vi "MoveSinglePIMotor.vi"(0 "System no.":i32=1 min=1 step=1, 1 "Axes to move":string[](array[string]), 2 "Move":dbl[](array[numeric]) format="%.6f", 5 "error in":errorcluster, 6 "Define home":bool, 7 "Move relative (-)":bool, 8 "Go home":bool, 9 "Move relative (+)":bool, 11 "Move absolute":bool, 12 "Stop refnum":refnum<vi>) -> (15 "Position":dbl[](array[numeric]) format="%.6f", 19 "error out":errorcluster)   [LabVIEW 2014]
doc: "This VI is runs in a loop until the stop button is pressed, the stop reference is TRUE or an error occures. It lets the operator set the velocity, move the connected axes to relative, absolute or to the home position, and reads the current position continuosly. The diagram shows how to combine the driver and support VIs for these tasks. Use the Help?Show Context Help menu sequence in the LabVIEW environment to display the Context Help window with the VI and control/indicator descriptions.\nRun \" XXXX_Configuration_Setup.vi\" (with XXXX being the PI product number of your system) prior to running this VI. \n\nValid for: C-843, C-843.PM, C-865, C-866, Mercury"
uses:
  C:/Users/Public/PI/GCSMergedLabVIEW/Low Level/General command.llb/Global2 (Array).vi
panel:
  in  "Clear":bool
  in  "stop":bool
  out "Conn. Axes":string[](array[string])
  # "Command move:"
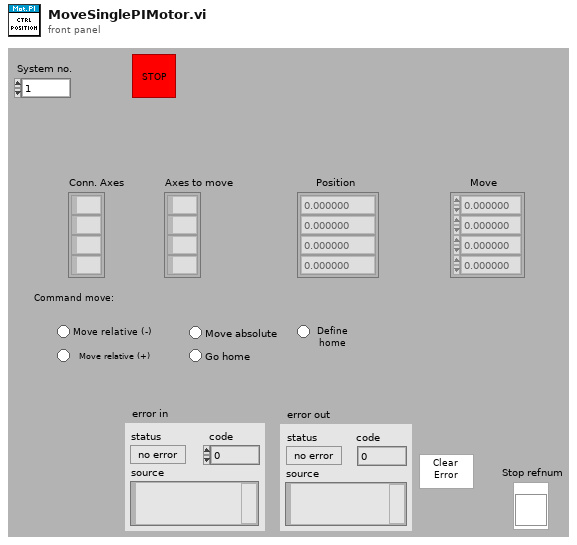
[diagram p1: front panel]
types:
  T1 = typedef "Controller names.ctl" = enum16{"None", "Analog", "C-702", "C-843", "C-843.PM", "C-844", "C-848", "C-865", "C-866", "C-867", "C-880", "C-884", "E-516", "E-517", "E-709", "E-710", "E-712", "E-725", "E-753", "E-755", "E-761", "E-816", "E-861", "E-870", "F-206", "HydraPollux", "M-840", "M-850", "M-8X0", "Mercury", "Mercury_GCS"}
  T2 = cluster{"Conn. axes":string[], "Controller name":T1}[]
  T3 = cluster{"Conn. axes":string[], "Controller name":T1}
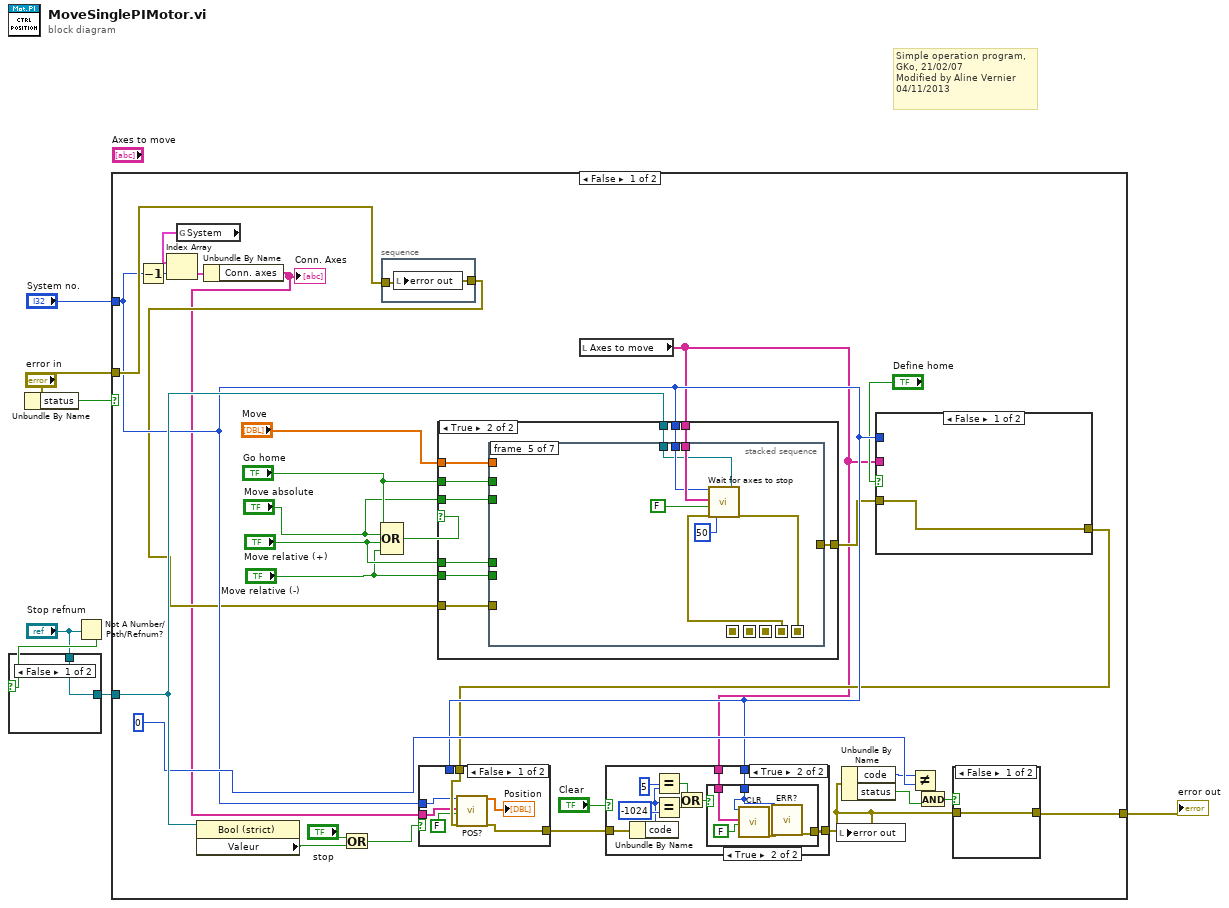
[diagram p0: block diagram]
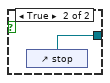
[diagram p2: hidden frame]
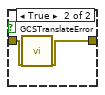
[diagram p3: hidden frame]
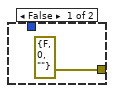
[diagram p5: hidden frame]
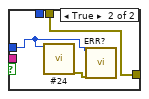
[diagram p6: hidden frame]
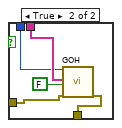
[diagram p9: hidden frame]
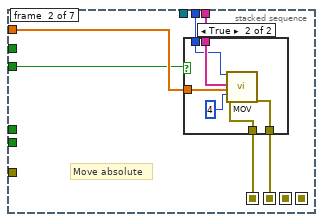
[diagram p10: hidden frame]
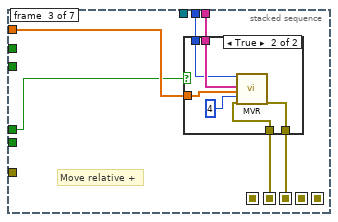
[diagram p12: hidden frame]
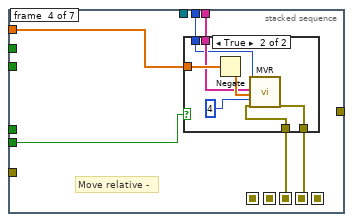
[diagram p14: hidden frame]
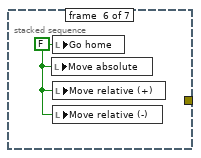
[diagram p16: hidden frame]
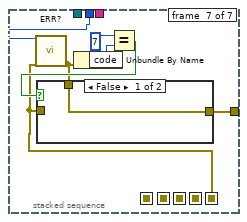
[diagram p17: hidden frame]
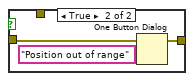
[diagram p18: hidden frame]
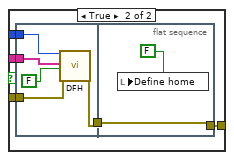
[diagram p19: hidden frame]
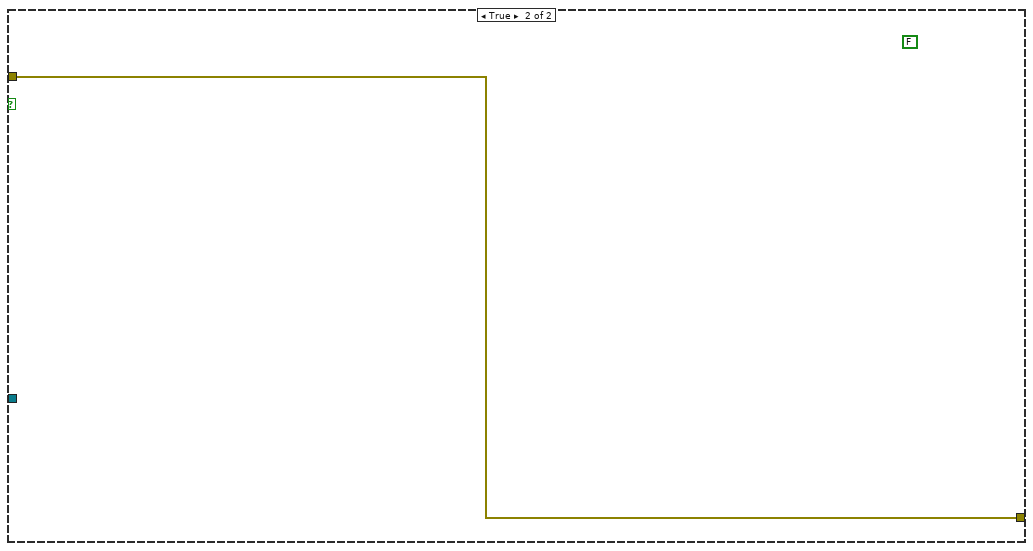
[diagram p20: hidden frame]
diagram:
  # "Simple operation program,\nGKo, 21/02/07\nModified by Aline Vernier\n04/11/2013"
  n1 = Unbundle By Name("error in") -> ("status"=w6:bool)
  n2 = Not A Number/Path/Refnum?(number/path/refnum="Stop refnum") -> (NaN/Path/Refnum?=w3:bool)
  n3 = case shown="False" w3 {
    tunnel: [w8 w9] -> w2
    tunnel: "Stop refnum" -> [w8 _]
    frame False {
    }
    frame True {
      n4 = control-ref of="stop"() -> (w9:refnum<vi>)
    }
  }
  n5 = case shown="False" w6 {
    tunnel: [w39 w163] -> w5
    tunnel: "error in" -> [w38 w163]
    tunnel: "System no." -> [w35 _]
    tunnel: w2 -> [w37 _]
    frame False {
      n6 = Decrement(x=w35) -> (x-1=w34:i32)
      n7 = global read "Global2 (Array).vi" "System"() -> (w33:T2)
      n8 = Index Array(array=w33, index=w34) -> (element=w32:T3)
      n9 = property class="Bool (strict)"(reference=w37) -> ("Valeur"=w26:bool)  [unwired: 1 in, 2 out]
      n10 = Unbundle By Name(w32) -> ("Conn. axes"=w11:string[])
      "Conn. Axes" <- w11
      n11 = Or(x="stop", y=w26) -> (x .or. y?=w12:bool)
      n12 = Compound Arithmetic op=OR("Go home", "Move absolute", "Move relative (+)", "Move relative (-)") -> (w14:bool)
      n13 = stacked-sequence {
        tunnel: w38 -> [w162]
        tunnel: [w162] -> w31
        frame #0 {
          n14 = local write "error out"(w162) -> ()
        }
      }
      n15 = local read "Axes to move"() -> (w13:string[])
      n16 = case shown="True" w14 {
        tunnel: "Go home" -> [_ w79]
        tunnel: w35 -> [_ w78]
        tunnel: w13 -> [_ w77]
        tunnel: "Move" -> [_ w76]
        tunnel: [w69 w75] -> w25
        tunnel: w37 -> [_ w74]
        tunnel: "Move absolute" -> [_ w73]
        tunnel: "Move relative (+)" -> [_ w72]
        tunnel: w31 -> [w69 w71]
        tunnel: "Move relative (-)" -> [_ w70]
        frame False {
        }
        frame True {
          n17 = stacked-sequence {
            seq-local: [w81 _ _ _ _ _ _] -> [_ w94 _ _ _ _ _]
            seq-local: [_ w92 _ _ _ _ _] -> [_ _ w105 _ _ _ _]
            seq-local: [_ _ w106 _ _ _ _] -> [_ _ _ w119 _ _ _]
            seq-local: [_ _ _ w118 _ _ _] -> [_ _ _ _ w137 _ _]
            seq-local: [_ _ _ _ w136 _ _] -> [_ _ _ _ _ _ w141]
            tunnel: w79 -> [w84 _ _ _ _ _ _]
            tunnel: w78 -> [w83 w96 w109 w122 w132 _ w142]
            tunnel: w77 -> [w82 w95 w108 w121 w133 _ _]
            tunnel: w76 -> [_ w93 w107 w120 _ _ _]
            tunnel: [_ _ _ _ _ _ w143] -> w75
            tunnel: w74 -> [_ _ _ _ w131 _ _]
            tunnel: w73 -> [_ w91 _ _ _ _ _]
            tunnel: w72 -> [_ _ w104 _ _ _ _]
            tunnel: w71 -> [w80 _ _ _ _ _ _]
            tunnel: w70 -> [_ _ _ w117 _ _ _]
            frame #0 {
              n18 = case shown="False" w84 {
                tunnel: w83 -> [_ w86]
                tunnel: w82 -> [_ w90]
                tunnel: [w85 w87] -> w81
                tunnel: w80 -> [w85 w88]
                frame False {
                }
                frame True {
                  n19 = call "GOH.vi"("System no."=w86, "GOH axes"=w90, "All axes?"=FALSE, "error in"=w88) -> ("error out"=w87:errorcluster)  [unwired: 15 in]
                }
              }
            }
            frame #1 {
              # "Move absolute"
              n20 = case shown="True" w91 {
                tunnel: w96 -> [_ w100]
                tunnel: w95 -> [_ w101]
                tunnel: w94 -> [w97 w102]
                tunnel: w93 -> [_ w98]
                tunnel: [w97 w99] -> w92
                frame False {
                }
                frame True {
                  n21 = call "MOV.vi"("System no."=w100, "Axes to move"=w101, "Position values"=w98, "No.of digits"=i16 4, "error in"=w102) -> ("error out"=w99:errorcluster)  [unwired: 14 in]
                }
              }
            }
            frame #2 {
              # "Move relative +"
              n22 = case shown="True" w104 {
                tunnel: w109 -> [_ w113]
                tunnel: w108 -> [_ w114]
                tunnel: w107 -> [_ w115]
                tunnel: [w110 w111] -> w106
                tunnel: w105 -> [w110 w112]
                frame False {
                }
                frame True {
                  n23 = call "MVR.vi"("System no."=w113, "Axes to move"=w114, "Position values"=w115, "No.of digits"=i16 4, "error in"=w112) -> ("error out"=w111:errorcluster)  [unwired: 14 in]
                }
              }
            }
            frame #3 {
              # "Move relative -"
              n24 = case shown="True" w117 {
                tunnel: w122 -> [_ w126]
                tunnel: w121 -> [_ w127]
                tunnel: w120 -> [_ w130]
                tunnel: w119 -> [w123 w125]
                tunnel: [w123 w124] -> w118
                frame False {
                }
                frame True {
                  n25 = Negate(x=w130) -> (-x=w128:dbl[])
                  n26 = call "MVR.vi"("System no."=w126, "Axes to move"=w127, "Position values"=w128, "No.of digits"=i16 4, "error in"=w125) -> ("error out"=w124:errorcluster)  [unwired: 14 in]
                }
              }
            }
            frame #4 {
              n27 = call "Wait for axes to stop.vi"("System no."=w132, "Axes to wait for"=w133, "With status bit polling?"=FALSE, "error in"=w137, "Polling cycle time, ms"=u32 50, "Stop refnum"=w131) -> ("error out"=w136:errorcluster)  [unwired: 12 in, 1 out]
            }
            frame #5 {
              w138 = FALSE ("Go home")
              n28 = local write "Move absolute"(w138) -> ()
              n29 = local write "Go home"(w138) -> ()
              n30 = local write "Move relative (+)"(w138) -> ()
              n31 = local write "Move relative (-)"(w138) -> ()
            }
            frame #6 {
              n32 = call "ERR?.vi"("System no."=w142, "error in"=w141) -> ("error out"=w140:errorcluster)  [unwired: 16 in, 1 out]
              n33 = Unbundle By Name(w140) -> ("code"=w139:i32)
              n34 = Equal?(x=7 ("y"), y=w139) -> (x = y?=w144:bool)
              n35 = case shown="False" w144 {
                tunnel: [w146 w147] -> w143
                tunnel: w141 -> [_ w147]
                tunnel: w140 -> [w146 _]
                frame False {
                }
                frame True {
                  n36 = One Button Dialog(message="Position out of range") -> ()  [unwired: 1 in, 1 out]
                }
              }
            }
          }
        }
      }
      n37 = case shown="False" "Define home" {
        tunnel: w35 -> [_ w154]
        tunnel: w13 -> [_ w153]
        tunnel: w25 -> [w149 w152]
        tunnel: [w149 w151] -> w24
        frame False {
        }
        frame True {
          n38 = flat-sequence {
            tunnel: w154 -> [w159]
            tunnel: w153 -> [w158]
            tunnel: w152 -> [w156]
            tunnel: [w155] -> w150
            tunnel: [w161] -> w151
            tunnel: w150 -> [w161]
            frame #0 {
              n39 = call "DFH.vi"("System no."=w159, "DFH axes"=w158, "All axes?"=FALSE, "error in"=w156) -> ("error out"=w155:errorcluster)  [unwired: 15 in]
            }
            frame #1 {
              n40 = local write "Define home"(FALSE ("All axes?")) -> ()
            }
          }
        }
      }
      n41 = case shown="False" w12 {
        tunnel: w35 -> [w60 w67]
        tunnel: w35 -> [_ _]
        tunnel: w24 -> [w63 w68]
        tunnel: [w64 w68] -> w22
        tunnel: w11 -> [w61 _]
        frame False {
          n42 = call "POS?.vi"("System no."=w60, "Axes to query"=w61, "All axes?"=FALSE, "error in"=w63) -> ("Position"=→"Position":dbl[], "error out"=w64:errorcluster)  [unwired: 14 in]
        }
        frame True {
          n43 = call "#24.vi"("System no."=w67) -> ("error out"=w66:errorcluster)  [unwired: 18 in]
          n44 = call "ERR?.vi"("System no."=w67, "error in"=w66) -> ()  [unwired: 16 in, 2 out]
        }
      }
      n45 = case shown="True" "Clear" {
        tunnel: [w43 w46] -> w18
        tunnel: w22 -> [w43 w50]
        tunnel: w35 -> [_ w45]
        tunnel: w13 -> [_ w44]
        frame False {
        }
        frame True {
          n46 = Unbundle By Name(w50) -> ("code"=w51:i32)
          n47 = Equal?(x=5 ("y"), y=w51) -> (x = y?=w49:bool)
          n48 = Equal?(x=w51, y=-1024) -> (x = y?=w47:bool)
          n49 = Or(x=w49, y=w47) -> (x .or. y?=w48:bool)
          n50 = case shown="True" w48 {
            tunnel: [errorcluster {"status"=FALSE, "code"=0, "source"=""} ("error out") w55] -> w46
            tunnel: w45 -> [_ w58]
            tunnel: w44 -> [_ w57]
            frame False {
            }
            frame True {
              n51 = call "CLR.vi"("System no."=w58, "CLR axes"=w57, "All axes?"=FALSE) -> ("error out"=w59:errorcluster)  [unwired: 16 in]
              n52 = call "ERR?.vi"("System no."=w58, "error in"=w59) -> ("error out"=w55:errorcluster)  [unwired: 16 in, 1 out]
            }
          }
        }
      }
      n53 = local write "error out"(w18) -> ()
      n54 = Unbundle By Name(w18) -> ("code"=w21:i32, "status"=w17:bool)
      n55 = Not Equal?(x=w21, y=0 ("code")) -> (x != y?=w20:bool)
      n56 = And(x=w20, y=w17) -> (x .and. y?=w19:bool)
      n57 = case shown="False" w19 {
        tunnel: w18 -> [w40 w42]
        tunnel: [w40 w41] -> w39
        frame False {
        }
        frame True {
          n58 = call "GCSTranslateError.vi"("error in"=w42) -> ("error out"=w41:errorcluster)  [unwired: 16 in, 2 out]
        }
      }
    }
    frame True {
      (unwired) FALSE ("stop")
    }
  }
  "error out" <- w5
